vi "Write_raw_block_header.vi"(0 "No of LDA samples":i32, 2 "Block Timings":T1, 3 "No of PWA samples":i32, 4 "Add to Block Header":string) -> (5 "Output string":string)   [LabVIEW 2017]
uses:
  Controls/Block_start_and_end.ctl
  Globals/Plug_in_data_global.vi
  Globals/Meas_global.vi
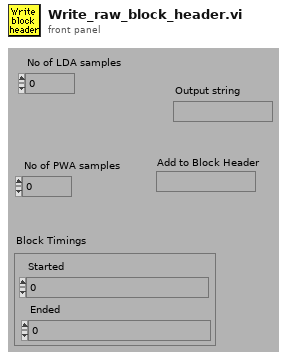
[diagram p1: front panel]
types:
  T1 = typedef "Block_start_and_end.ctl" = cluster{"Started":dbl, "Ended":dbl}
  T2 = typedef "Ch_description_ADAM.ctl" = cluster{"Ch Name":string, "Type":T3, "Function":T4, "Ch State":T5, "Calibration type":T6, "A":dbl, "B":dbl, "C":dbl, "D":dbl, "Comments":string, "Address":T7, "String":string, "Duty":u16}
  T3 = typedef "Module_type_ADAM.ctl" = string
  T4 = typedef "Function_ADAM.ctl" = enum16{"Analogue Input", "Digital Input", "Event counter", "Event rate", "Analogue Output", "Digital Output", "Relay Output"}
  T5 = typedef "Channel_State.ctl" = enum16{"On", "Off", "Always On", "Always Off"}
  T6 = typedef "Calib_type_ADAM.ctl" = string
  T7 = typedef "Address.ctl" = cluster{"Main":i32, "Ch.":i32, "Sub":i32, "Port Name":string}
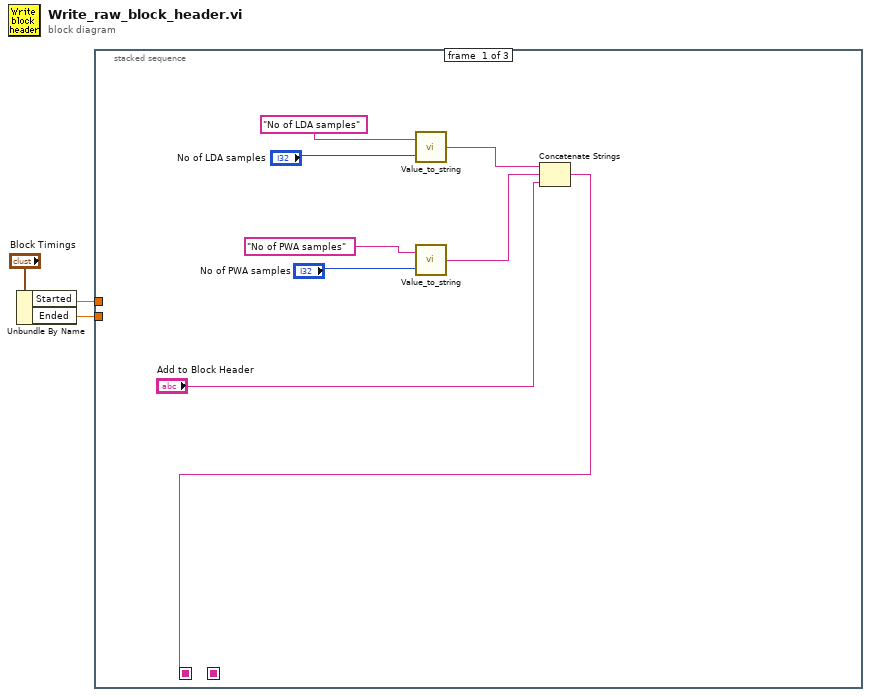
[diagram p0: block diagram]
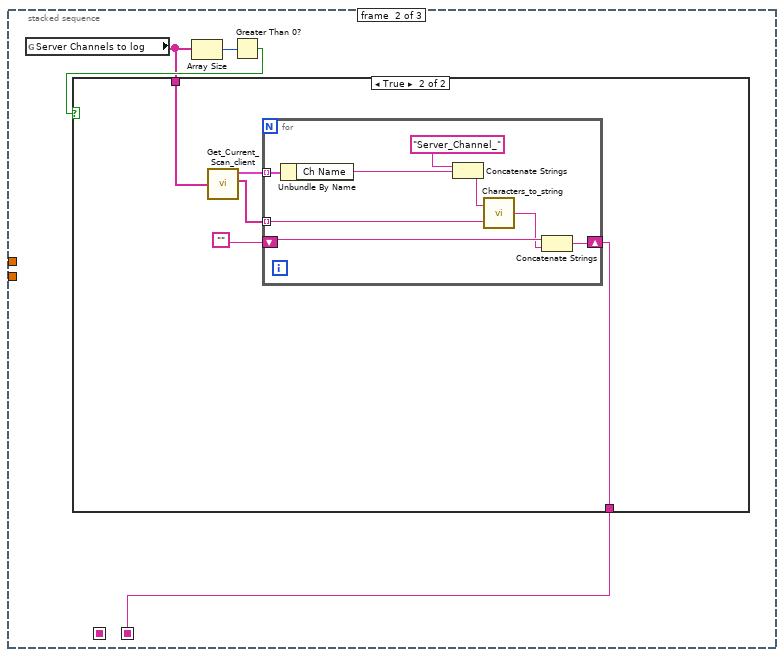
[diagram p2: hidden frame]
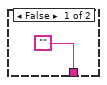
[diagram p3: hidden frame]
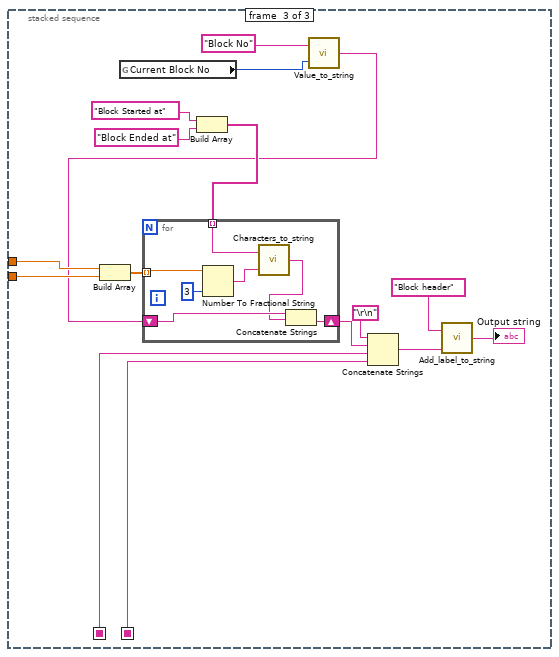
[diagram p4: hidden frame]
diagram:
  n1 = Unbundle By Name("Block Timings") -> ("Started"=w2:dbl, "Ended"=w1:dbl)
  n2 = stacked-sequence {
    seq-local: [w8 _ _] -> [_ _ w44]
    seq-local: [_ w12 _] -> [_ _ w31]
    tunnel: w2 -> [_ _ w37]
    tunnel: w1 -> [_ _ w36]
    frame #0 {
      n3 = call "Value_to_string.vi"("Value"="No of LDA samples", "Label for value"="No of LDA samples") -> ("Output string"=w9:string)  [unwired: 1 in]
      n4 = call "Value_to_string.vi"("Value"="No of PWA samples", "Label for value"="No of PWA samples") -> ("Output string"=w5:string)  [unwired: 1 in]
      n5 = Concatenate Strings(w9, w5, "Add to Block Header") -> (w8:string)
    }
    frame #1 {
      n6 = global read "Plug_in_data_global.vi" "Server Channels to log"() -> (w13:string[])
      n7 = Array Size(array=w13) -> (size(s)=w15:i32)
      n8 = Greater Than 0?(x=w15) -> (x > 0?=w14:bool)
      n9 = case shown="True" w14 {
        tunnel: w13 -> [_ w20]
        tunnel: ["" w17] -> w12
        frame False {
        }
        frame True {
          n10 = call "Get_Current_Scan_client.vi"("ADAM Ch Names"=w20) -> ("Ch Description Array"=w19:T2[], "String values"=w18:string[])  [unwired: 2 out]
          n11 = for {
            shift-right: [w28] -> w17
            shift-left: "" -> [w27]
            tunnel: w19 -> [w24] mode=indexing
            tunnel: w18 -> [w22] mode=indexing
            n12 = Unbundle By Name(w24) -> ("Ch Name"=w23:string)
            n13 = Concatenate Strings("Server_Channel_" ("string"), w23) -> (w25:string)
            n14 = call "Characters_to_string.vi"("Characters to write"=w22, "Label for characters"=w25) -> ("Output string"=w26:string)
            n15 = Concatenate Strings(w27, w26) -> (w28:string)
          }
        }
      }
    }
    frame #2 {
      n16 = Build Array(w37, w36) -> (w38:dbl[])
      n17 = global read "Meas_global.vi" "Current Block No"() -> (w30:i32)
      n18 = Build Array("Block Started at", "Block Ended at") -> (w40:string[])
      n19 = call "Value_to_string.vi"("Value"=w30, "Label for value"="Block No") -> ("Output string"=w34:string)  [unwired: 1 in]
      n20 = for {
        tunnel: w40 -> [w52] mode=indexing
        shift-right: [w49] -> w42
        shift-left: w34 -> [w51]
        tunnel: w38 -> [w47] mode=indexing
        n21 = Number To Fractional String(number=w47, precision (6)=i16 3) -> (F-format string=w46:string)  [unwired: 2 out]
        n22 = call "Characters_to_string.vi"("Characters to write"=w46, "Label for characters"=w52) -> ("Output string"=w50:string)
        n23 = Concatenate Strings(w51, w50) -> (w49:string)
      }
      n24 = Concatenate Strings("\r\n", w42, w44, w31) -> (w43:string)
      n25 = call "Add_label_to_string.vi"("String to write"=w43, "File Label"="Block header") -> ("Output string"=→"Output string":string)
    }
  }
